vi "Configure Multi Eval Meas List Segment PUSCH Allocation.vi"(0 "VISA resource name":refnum<visa-resource-name>, 1 "Allocation (1)":T1=1, 2 "No Symbols (4)":i32=4, 3 "Auto Detect (Off)":bool, 5 "Instance (1)":T3=1, 7 "Segment (1)":i32=1, 8 "Modulation Scheme (Pi/2-BPSK)":i32(ring) items=["Pi/2-BPSK", "QPSK", "16-QAM", "64-QAM", "256-QAM", "Pi/2-BPSK with shaping"], 9 "CC (1)":T2=1, 10 "Start RB (0)":i32, 11 "error in (no error)":errorcluster, 12 "Mapping Type (A)":i32(ring) items=["A", "B"], 13 "Start Symbol (0)":i32, 14 "No RBs (1)":i32=1) -> (4 "VISA resource name out":refnum<visa-resource-name>, 15 "error out":errorcluster)   [LabVIEW 2020, in "Rohde&Schwarz CMWXP NR FR1 Measurement.lvlib"]
doc: "Specifies settings related to the PUSCH allocation, for carrier <cc>, allocation <a> in segment <no>.\n\nAttribute:\nRSCMWXPNRFR1M_ATTR_MULTI_EVAL_MEAS_LIST_SEGMENT_PUSCH_ALLOCATION\n\nRemote-control command:\nCONFigure:NRSub:MEAS<i>:LIST:SEGMent<no>[:CC<cc>]:ALLocation<a>:PUSCh"
uses:
  <instrlib>/Rohde&Schwarz CMWXP NR FR1 Measurement/Rohde&Schwarz CMWXP NR FR1 Measurement.lvlib
  <instrlib>/Rohde&Schwarz CMWXP NR FR1 Measurement/Private/_Instance.ctl
  <instrlib>/Rohde&Schwarz CMWXP NR FR1 Measurement/Private/_Carrier Component.ctl
  <instrlib>/Rohde&Schwarz CMWXP NR FR1 Measurement/Private/_Allocation.ctl
  <instrlib>/Rohde&Schwarz CMWXP NR FR1 Measurement/Private/rsidr_core.llb/rsidr_core.lvlib
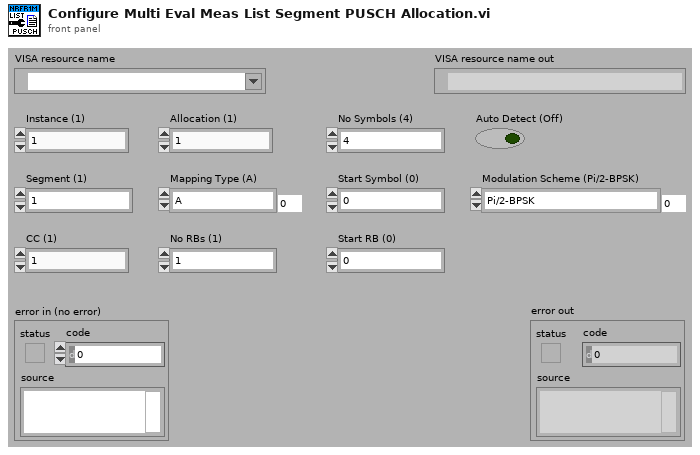
[diagram p1: front panel]
types:
  T1 = typedef "Rohde&Schwarz CMWXP NR FR1 Measurement.lvlib/_Allocation.ctl" = i32
  T2 = typedef "Rohde&Schwarz CMWXP NR FR1 Measurement.lvlib/_Carrier Component.ctl" = i32
  T3 = typedef "Rohde&Schwarz CMWXP NR FR1 Measurement.lvlib/_Instance.ctl" = i32
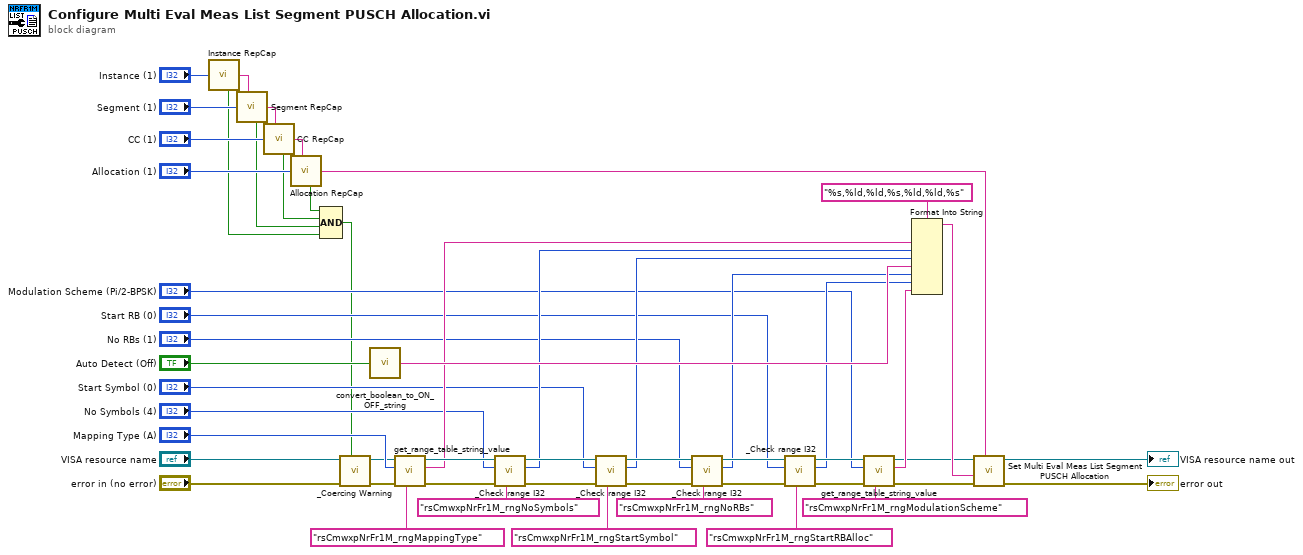
[diagram p0: block diagram]
diagram:
  n1 = call <instrlib>:"Instance RepCap.vi"("Instance In"="Instance (1)") -> ("In Range?"=w8:bool, "RepCap Identifier Out"=w46:string)  [unwired: 1 in]
  n2 = call <instrlib>:"Segment RepCap.vi"("Segment In"="Segment (1)", "RepCap String In (\"\")"=w46) -> ("In Range?"=w9:bool, "RepCap Identifier Out"=w47:string)
  n3 = call <instrlib>:"CC RepCap.vi"("CC In"="CC (1)", "RepCap String In (\"\")"=w47) -> ("In Range?"=w7:bool, "RepCap Identifier Out"=w50:string)
  n4 = call <instrlib>:"Allocation RepCap.vi"("Allocation In"="Allocation (1)", "RepCap String In (\"\")"=w50) -> ("In Range?"=w6:bool, "RepCap Identifier Out"=w44:string)
  n5 = Compound Arithmetic op=AND(w6, w7, w9, w8) -> (w1:bool)
  n6 = call <instrlib>:"_Coercing Warning.vi"("In Range?"=w1, "error in (no error)"="error in (no error)", "VISA resource name"="VISA resource name") -> ("error out"=w3:errorcluster, "VISA resource name out"=w2:refnum<visa-resource-name>)  [unwired: 7 in]
  n7 = call <instrlib>:"convert_boolean_to_ON_OFF_string.vi"("boolean value in"="Auto Detect (Off)") -> ("string value out"=w41:string)  [unwired: 4 in]
  n8 = call <instrlib>:"get_range_table_string_value.vi"("Range Table ID in"="rsCmwxpNrFr1M_rngMappingType", "error in"=w3, "I32 input"="Mapping Type (A)", "VISA resource name"=w2) -> ("error out"=w40:errorcluster, "String Value out"=w29:string, "VISA resource name out"=w39:refnum<visa-resource-name>)  [unwired: 5 in]
  n9 = call <instrlib>:"_Check range I32.vi"("Range Table Identifier"="rsCmwxpNrFr1M_rngNoSymbols", "error in (no error)"=w40, "I32 Value In"="No Symbols (4)", "VISA resource name"=w39) -> ("error out"=w38:errorcluster, "I32 Value Out"=w28:i32, "VISA resource name out"=w37:refnum<visa-resource-name>)  [unwired: 5 in]
  n10 = call <instrlib>:"_Check range I32.vi"("Range Table Identifier"="rsCmwxpNrFr1M_rngStartSymbol", "error in (no error)"=w38, "I32 Value In"="Start Symbol (0)", "VISA resource name"=w37) -> ("error out"=w36:errorcluster, "I32 Value Out"=w27:i32, "VISA resource name out"=w35:refnum<visa-resource-name>)  [unwired: 5 in]
  n11 = call <instrlib>:"_Check range I32.vi"("Range Table Identifier"="rsCmwxpNrFr1M_rngNoRBs", "error in (no error)"=w36, "I32 Value In"="No RBs (1)", "VISA resource name"=w35) -> ("error out"=w34:errorcluster, "I32 Value Out"=w26:i32, "VISA resource name out"=w33:refnum<visa-resource-name>)  [unwired: 5 in]
  n12 = call <instrlib>:"_Check range I32.vi"("Range Table Identifier"="rsCmwxpNrFr1M_rngStartRBAlloc", "error in (no error)"=w34, "I32 Value In"="Start RB (0)", "VISA resource name"=w33) -> ("error out"=w32:errorcluster, "I32 Value Out"=w25:i32, "VISA resource name out"=w31:refnum<visa-resource-name>)  [unwired: 5 in]
  n13 = call <instrlib>:"get_range_table_string_value.vi"("Range Table ID in"="rsCmwxpNrFr1M_rngModulationScheme", "error in"=w32, "I32 input"="Modulation Scheme (Pi/2-BPSK)", "VISA resource name"=w31) -> ("error out"=w23:errorcluster, "String Value out"=w24:string, "VISA resource name out"=w10:refnum<visa-resource-name>)  [unwired: 5 in]
  n14 = Format Into String(format string="%s,%ld,%ld,%s,%ld,%ld,%s", w29, w28, w27, w41, w26, w25, w24) -> (resulting string=w11:string)  [unwired: 2 in, 1 out]
  n15 = call "Set Multi Eval Meas List Segment PUSCH Allocation"("Repeated Capabilities"=w44, "error in (no error)"=w23, "Multi Eval Meas List Segment PUSCH Allocation ()"=w11, "instrument handle"=w10) -> ("error out"=→"error out":errorcluster, "instrument handle out"=→"VISA resource name out":refnum<visa-resource-name>)  [unwired: 6 in]
